vi "TestExec.Client, Equipment List Items.vi"(7 "Module Q Name":string, 8 "error in":errorcluster, 10 "Eq List":T1[](array[typedef]), 11 "Q In":refnum<queue>) -> (0 "error out":errorcluster)   [LabVIEW 2019]
uses:
  <vilib>/KATE/Queues/Q.Element.ctl
  Results/Result XML/TestResult.HW Item.ctl
  <vilib>/KATE/Queues/Queue Utils.lvlib
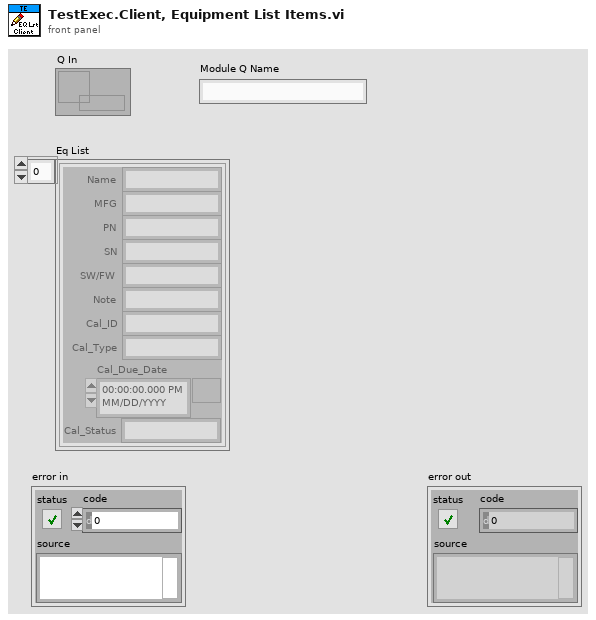
[diagram p1: front panel]
types:
  T1 = typedef "TestResult.HW Item.ctl" = cluster{"Name":string, "MFG":string, "PN":string, "SN":string, "SW/FW":string, "Note":string, "Cal_ID":string, "Cal_Type":string, "Cal_Due_Date":timestamp, "Cal_Status":string}
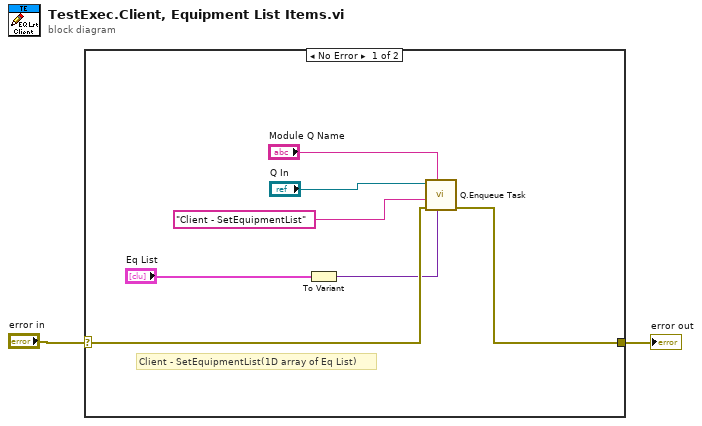
[diagram p0: block diagram]
diagram:
  n1 = case shown="No Error" "error in" {
    selector: "error in" -> [w6 w10]
    tunnel: [w7 w10] -> w1
    frame No Error {
      # "Client - SetEquipmentList(1D array of Eq List)"
      n2 = To Variant(anything="Eq List") -> (Variant=w5:variant)
      n3 = call <vilib>:"Q.Enqueue Task.vi"("Data1"=w5, "Q Name"="Module Q Name", "Error In"=w6, "Task Name"="Client - SetEquipmentList" ("Cmd"), "Q In"="Q In") -> ("error out"=w7:errorcluster)  [unwired: 5 in, 1 out]
    }
    frame Error {
    }
  }
  "error out" <- w1
